vi "Variables.vi"(10 "Ele_At_Pos":bool, 11 "Ref_Num":T24) -> (3 "Var":T1)   [LabVIEW 2014]
uses:
  <vilib>/Rock Robotics/WPI/Joystick/WPI_JoystickDevRef.ctl
  <vilib>/Rock Robotics/WPI/Joystick/WPI_JoystickDeviceEnum.ctl
  <vilib>/Rock Robotics/WPI/RobotDrive/WPI_RobotDriveDevRef.ctl
  <vilib>/Rock Robotics/WPI/MotorControl/WPI_MotorControlDeviceRef.ctl
  <vilib>/Rock Robotics/WPI/MotorControl/WPI_MotorControlType.ctl
  <vilib>/Rock Robotics/SystemInterfaces/Typedef/FPGA_TypedefDigitalModule.ctl
  <vilib>/Rock Robotics/SystemInterfaces/DIO/FPGA_DIOPWMChannel.ctl
  <vilib>/Rock Robotics/WPI/PWM/WPI_PWMDeadband.ctl
  <vilib>/Rock Robotics/WPI/CAN/Jaguar/SubVIs/WPI_CANJaguar_ControlMode.ctl
  <vilib>/Rock Robotics/WPI/CAN/TalonSRX/WPI_CANTalonSRX_APIControlMode.ctl
  <vilib>/Rock Robotics/WPI/PWM/WPI_PWMTransform_ConPane.ctl
  <vilib>/Rock Robotics/WPI/Encoder/WPI_EncoderDevRef.ctl
  <vilib>/Rock Robotics/SystemInterfaces/Encoder/FPGA_EncoderIdx.ctl
  <vilib>/Rock Robotics/SystemInterfaces/Counter/FPGA_CounterCtrSystemIndex.ctl
  <vilib>/Rock Robotics/WPI/Encoder/WPI_EncoderType.ctl
  <vilib>/Rock Robotics/WPI/AnalogChannel/WPI_AnalogChannelDevRef.ctl
  <vilib>/Rock Robotics/SystemInterfaces/Typedef/FPGA_TypedefAnalogModule.ctl
  <vilib>/Rock Robotics/SystemInterfaces/AI/FPGA_AIChannel.ctl
  <vilib>/Rock Robotics/WPI/Gyro/WPI_GyroDevRef.ctl
  AdaIMU roboRIO/IMUDevRef.ctl
  <vilib>/Rock Robotics/SystemInterfaces/i2clib/i2c_bus.ctl
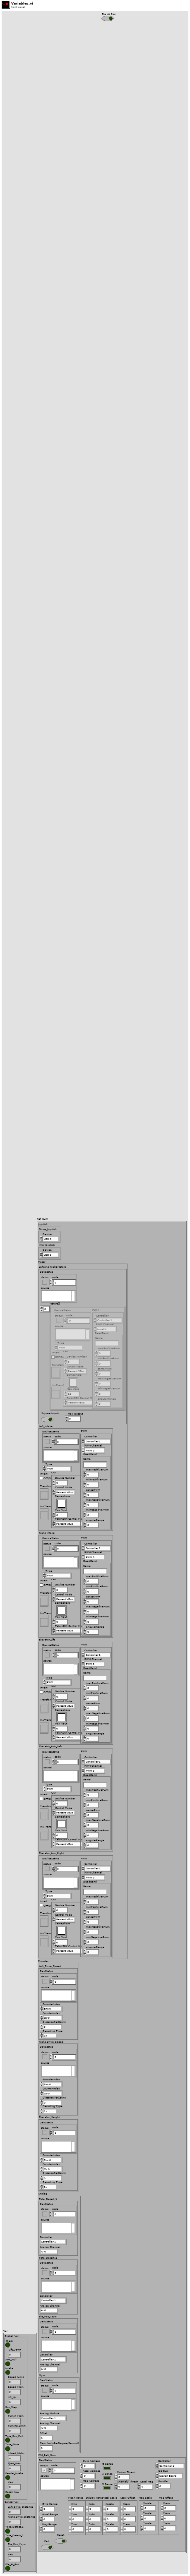
[diagram p1: front panel]
types:
  T1 = cluster{"Global_Var":cluster{" Eject":bool, " Lift_Down":dbl, "Arm_Pull":bool, "Intake":bool, "Speed_Limit":dbl, "Speed_Main":dbl, "Lift_Up":dbl, "Pos_Step":bool, "Turnin_Main":dbl, "Turning_Limit":dbl, "Tote_Pos_Exit":bool, "Tote_Store":bool, "Infeed_Motor":dbl, "Eject_Man":dbl, "Feeder_Intake":bool, "Yaw":dbl, "Reset_Yaw":bool}, "Sensor_Val":cluster{"Left_Drive_Distance":dbl, "Right_Drive_Distance":dbl, "Tote_Detect_1":bool, "Tote_Detect_2":bool, "Ele_Pos_Yoyo":dbl, "Yaw":dbl, "Ele_At_Pos":bool}}
  T2 = typedef "WPI_JoystickDevRef.ctl" = cluster{"Device":T3}
  T3 = typedef "WPI_JoystickDeviceEnum.ctl" = enum16{"USB 0", "USB 1", "USB 2", "USB 3", "USB 4", "USB 5"}
  T4 = typedef "WPI_RobotDriveDevRef.ctl" = cluster{"DevStatus":errorcluster, "Motors[]":T5[], "Square Inputs":bool, "Max Output":dbl}
  T5 = typedef "WPI_MotorControlDeviceRef.ctl" = cluster{"DeviceStatus":errorcluster, "Type":T6, "PWM":cluster{"Controller":T7, "PWM Channel":T8, "DeadBand":T9}, "CAN":cluster{"Device Number":u8, "Control Mode":T10, "Semaphore":T11, "Max Vout":dbl, "TalonSRX Control Mode":T12}, "Invert":bool, "TransformRef":T13, "InvTransformRef":T13}
  T6 = typedef "WPI_MotorControlType.ctl" = enum16{"PWM", "CAN", "CANTalonSRX"}
  T7 = typedef "FPGA_TypedefDigitalModule.ctl" = enum16{"Controller 1"}
  T8 = typedef "FPGA_DIOPWMChannel.ctl" = enum8{"PWM 0", "PWM 1", "PWM 2", "PWM 3", "PWM 4", "PWM 5", "PWM 6", "PWM 7", "PWM 8", "PWM 9", "PWM MXP 0", "PWM MXP 1", "PWM MXP 2", "PWM MXP 3", "PWM MXP 4", "PWM MXP 5", "PWM MXP 6", "PWM MXP 7", "PWM MXP 8", "PWM MXP 9", "Invalid"}
  T9 = typedef "WPI_PWMDeadband.ctl" = cluster{"Name":string, "maxPositivePwm":i32, "minPositivePwm":i32, "centerPwm":i32, "maxNegativePwm":i32, "minNegativePwm":i32, "angularRange":u16}
  T10 = typedef "WPI_CANJaguar_ControlMode.ctl" = enum8{"Percent VBus", "Current", "Speed", "Position", "Voltage"}
  T11 = typedef "Semaphore RefNum" = refnum<k1>
  T12 = typedef "WPI_CANTalonSRX_APIControlMode.ctl" = enum8{"Percent VBus", "Speed", "Position", "Slave", "Unchanged / Invalid"}
  T13 = typedef "WPI_PWMTransform_ConPane.ctl" = refnum<vi>
  T14 = typedef "WPI_EncoderDevRef.ctl" = cluster{"DevStatus":errorcluster, "EncoderIndex":T15, "CounterIndex":T16, "DistancePerCount":dbl, "Decoding Type":T17}
  T15 = typedef "FPGA_EncoderIdx.ctl" = enum8{"Enc 0", "Enc 1", "Enc 2", "Enc 3", "Enc 4", "Enc 5", "Enc 6", "Enc 7", "Invalid"}
  T16 = typedef "FPGA_CounterCtrSystemIndex.ctl" = enum8{"Ctr 0", "Ctr 1", "Ctr 2", "Ctr 3", "Ctr 4", "Ctr 5", "Ctr 6", "Ctr 7", "Invalid"}
  T17 = typedef "WPI_EncoderType.ctl" = enum16{"1x", "2x", "4x"}
  T18 = typedef "WPI_AnalogChannelDevRef.ctl" = cluster{"DevStatus":errorcluster, "Controller":T19, "Analog Channel":T20}
  T19 = typedef "FPGA_TypedefAnalogModule.ctl" = enum16{"Controller 1"}
  T20 = typedef "FPGA_AIChannel.ctl" = enum8{"AI 0", "AI 1", "AI 2", "AI 3", "AI MXP 0", "AI MXP 1", "AI MXP 2", "AI MXP 3", "Invalid"}
  T21 = typedef "WPI_GyroDevRef.ctl" = cluster{"DevStatus":errorcluster, "Analog Module":T19, "Analog Channel":T20, "Offset":dbl, "Gain (VoltsPerDegree/Second)":dbl}
  T22 = typedef "IMUDevRef.ctl" = cluster{"DevStatus":errorcluster, "Gyro Address":u8, "Gyro Range":u8, "Mean Rates":cluster{"Xmo":dbl, "Ymo":dbl, "Zmo":dbl}, "StdDev Rates":cluster{"Xsdo":dbl, "Ysdo":dbl, "Zsdo":dbl}, "Fast":bool, "Reset":bool, "Accel Address":u8, "Accel Range":u8, "Accel Scale":cluster{"Xscale":dbl, "Yscale":dbl, "Zscale":dbl}, "Mag Address":u8, "Mag Range":u8, "G Sense":bool, "A Sense":bool, "M Sense":bool, "Accel Offset":cluster{"Xzero":dbl, "Yzero":dbl, "Zzero":dbl}, "Motion Thresh":dbl, "Mag Scale":cluster{"Xscale":dbl, "Yscale":dbl, "Zscale":dbl}, "Mag Offset":cluster{"Xzero":dbl, "Yzero":dbl, "Zzero":dbl}, "I2C Bus":T23, "Handle":i32, "Controller":T7, "Anomaly Thresh":dbl, "Local Mag":dbl}
  T23 = typedef "i2c_bus.ctl" = enum16{"I2C On-Board", "I2C MXP", "Invalid"}
  T24 = cluster{"Joystick":cluster{"Drive_Joystick":T2, "Imp_Joystick":T2}, "Motor":cluster{"Left and Right Motors":T4, "Left_Intake":T5, "Right_Intake":T5, "Elevator_Lift":T5, "Elevator_Arm_Left":T5, "Elevator_Arm_Right":T5}, "Encoder":cluster{"Left_Drive_Speed":T14, "Right_Drive_Speed":T14, "Elevator_Height":T14}, "Analog":cluster{"Tote_Detect_1":T18, "Tote_Detect_2":T18, "Ele_Pos_Yoyo":T18, "Gyro":T21}, "IMU_Reft_Num":T22}
  T25 = cluster{" Eject":bool, " Lift_Down":dbl, "Arm_Pull":bool, "Intake":bool, "Speed_Limit":dbl, "Speed_Main":dbl, "Lift_Up":dbl, "Pos_Step":bool, "Turnin_Main":dbl, "Turning_Limit":dbl, "Tote_Pos_Exit":bool, "Tote_Store":bool, "Infeed_Motor":dbl, "Eject_Man":dbl, "Feeder_Intake":bool, "Yaw":dbl, "Reset_Yaw":bool}
  T26 = cluster{"Left_Drive_Distance":dbl, "Right_Drive_Distance":dbl, "Tote_Detect_1":bool, "Tote_Detect_2":bool, "Ele_Pos_Yoyo":dbl, "Yaw":dbl, "Ele_At_Pos":bool}
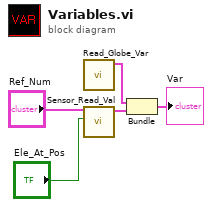
[diagram p0: block diagram]
diagram:
  n1 = call "Read_Globe_Var.vi"() -> ("Global_Var"=w3:T25)  [unwired: 11 in]
  n2 = call "Sensor_Read_Val.vi"("Ele_At_Pos"="Ele_At_Pos", "Ref_Num"="Ref_Num") -> ("Sensor_Val"=w4:T26)  [unwired: 9 in]
  n3 = Bundle("Global_Var"=w3, "Sensor_Val"=w4) -> (→"Var":T1)  [unwired: 1 in]
